vi "Update shutter GUI.vi"(8 "error in (no error)":errorcluster, 10 "shutter on/off":bool, 11 "AOTF in":refnum<class "Invivo_AOTF.lvclass">) -> (0 "error out":errorcluster, 3 "AOTF out":refnum<class "Invivo_AOTF.lvclass">)   [LabVIEW 2012, in "Invivo_AOTF.lvclass"]
uses:
  Invivo_AOTF.lvclass
  Invivo_AOTF.lvclass/Invivo_AOTF.ctl
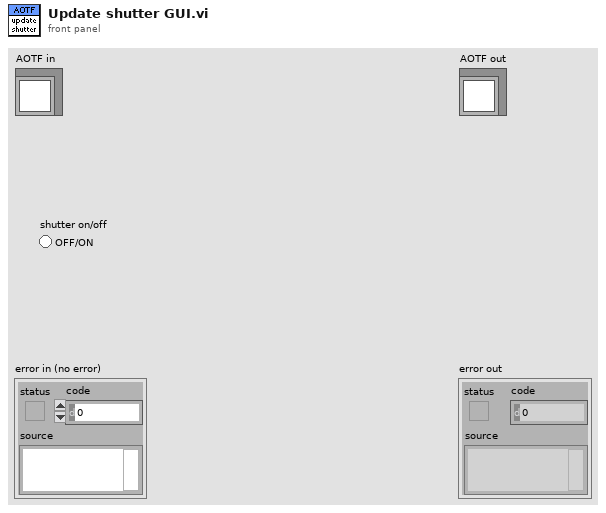
[diagram p1: front panel]
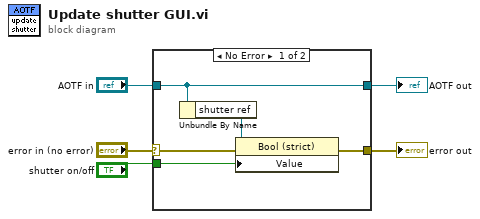
[diagram p0: block diagram]
diagram:
  n1 = case shown="No Error" "error in (no error)" {
    selector: "error in (no error)" -> [w8 w12]
    tunnel: [w7 w12] -> w4
    tunnel: [w10 w11] -> w2
    tunnel: "AOTF in" -> [w10 w11]
    tunnel: "shutter on/off" -> [w6 _]
    frame No Error {
      n2 = Unbundle By Name(w10) -> ("shutter ref"=w9:refnum<vi>)
      n3 = property class="Bool (strict)"(reference=w9, error in=w8, "Value"=w6) -> (error out=w7:errorcluster)  [unwired: 1 out]
    }
    frame Error {
    }
  }
  "error out" <- w4
  "AOTF out" <- w2
